vi "DDE2TCP_main.vi"() -> ()   [LabVIEW 2013]
uses:
  <vilib>/Utility/error.llb/DialogType.ctl
  _OpenG.lib/comparison.llb/Variant Changed__ogtk.vi
panel:
  in  "listen halted":bool caption="Listener gestoppt"
  in  "empty":refnum<k5>[](array[refnum]) caption="Leer"
  in  "empty 2":refnum<k5>[](array[refnum]) caption="Leer"
  out "Pfad":path
  out "String":string
  in  "Registerkarte":enum32{"MyDDE2TCP", "Data file", "Sim"}(tab)
  out "status":bool
  out "data":string="\r\n" caption="DDE Message"
  out "# of Connections":dbl caption="Client connections"
  in  "Port":u16=6341 caption="TCP Port"
  in  "stop":bool caption="Stopp"
  out "Azimuth":string caption="°"
  out "Elevation":string caption="°"
  out "Satellite Name":string
  out "Downlink Freq. Setpoint":string caption="Hz"
  out "Uplink Freq. Setpoint":string caption="Hz"
  out "Current JD [UTC]":dbl=2456800.0578935184 format="%#.15g"
  out "Unix time":dbl=1400757802.7173696 format="%#_13g"
  out "Time Stamp (UTC)":timestamp=timestamp(3483602602.7173696 s since 1904-01-01) format="%^<%.3X   %x>T"
  out "Current Modified JD [UTC]":dbl=2456800.0578935184 format="%#.15g"
  in  "Sampling interval":u32=250 caption="[ms]"
  in  "Save Controls":bool
  out "Tracking data":string
  out "Path of the saved data":path
  out "concatenated string":string
  in  "Radio Buttons":enum32{"Realtime", "Simulated time"}(radio)
  in  "Simulated time":timestamp
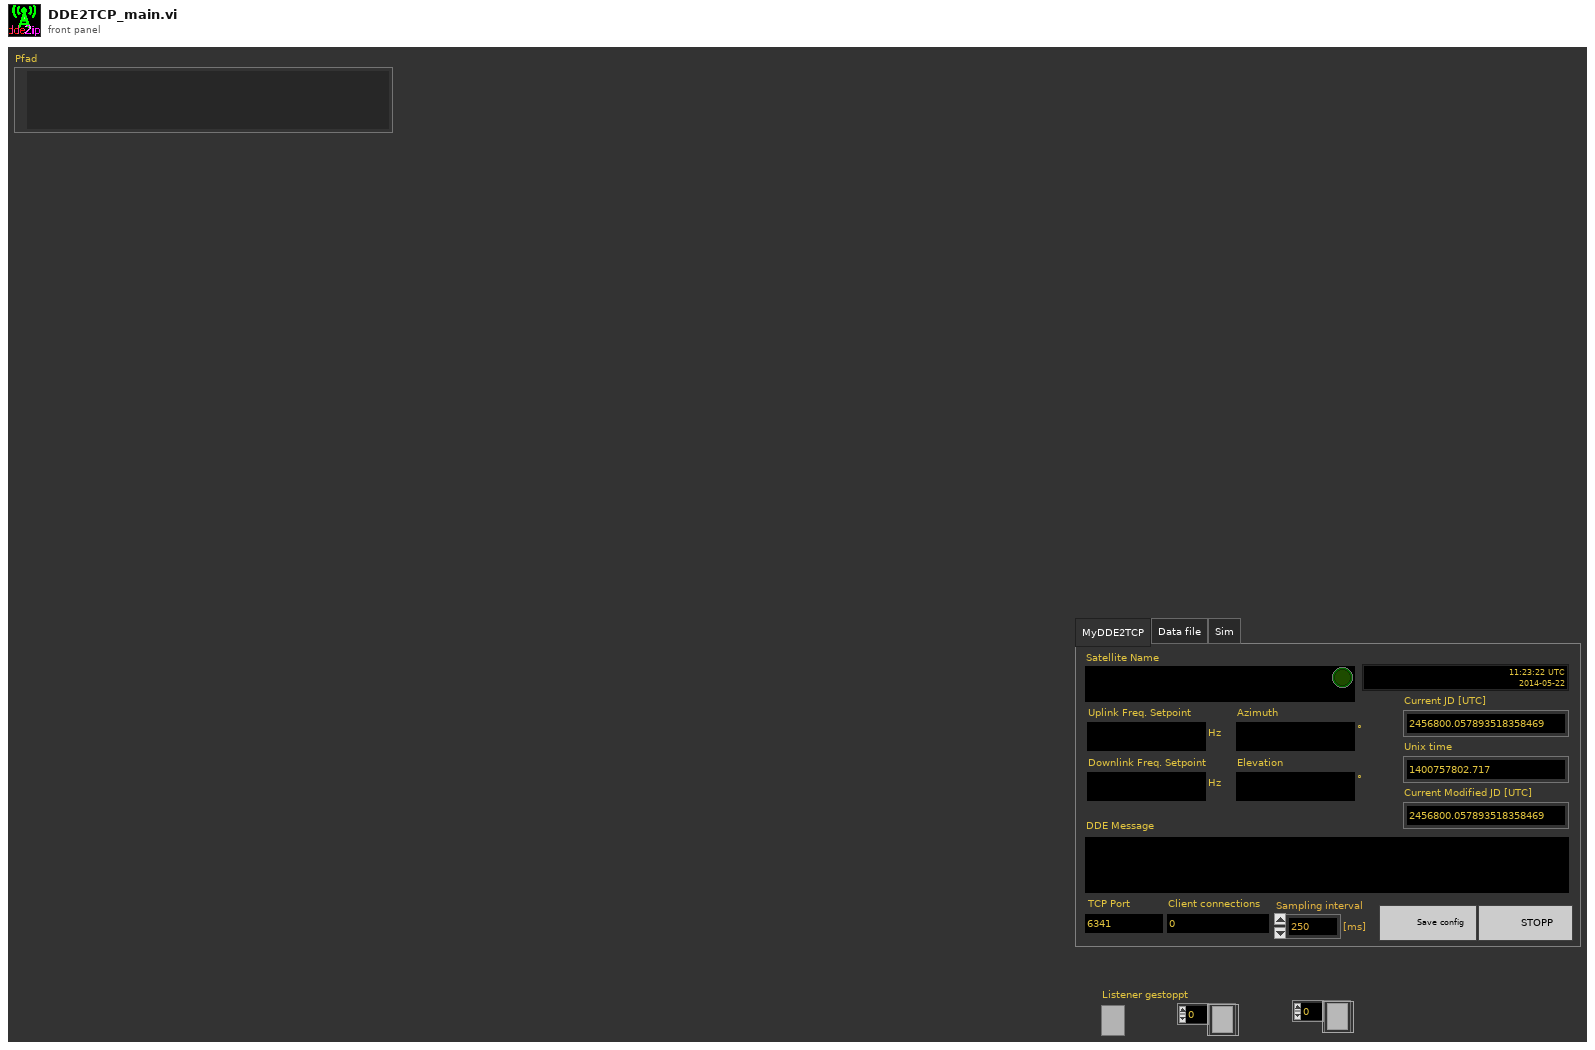
[diagram p1: front panel]
types:
  T1 = typedef "DialogType.ctl" = u16
  T2 = typedef "LVDateTimeRec.ctl" = cluster{"fractional second":dbl, "second":i32, "minute":i32, "hour":i32, "day of month":i32, "month":i32, "year":i32, "day of week":i32, "day of year":i32, "DST":i32}
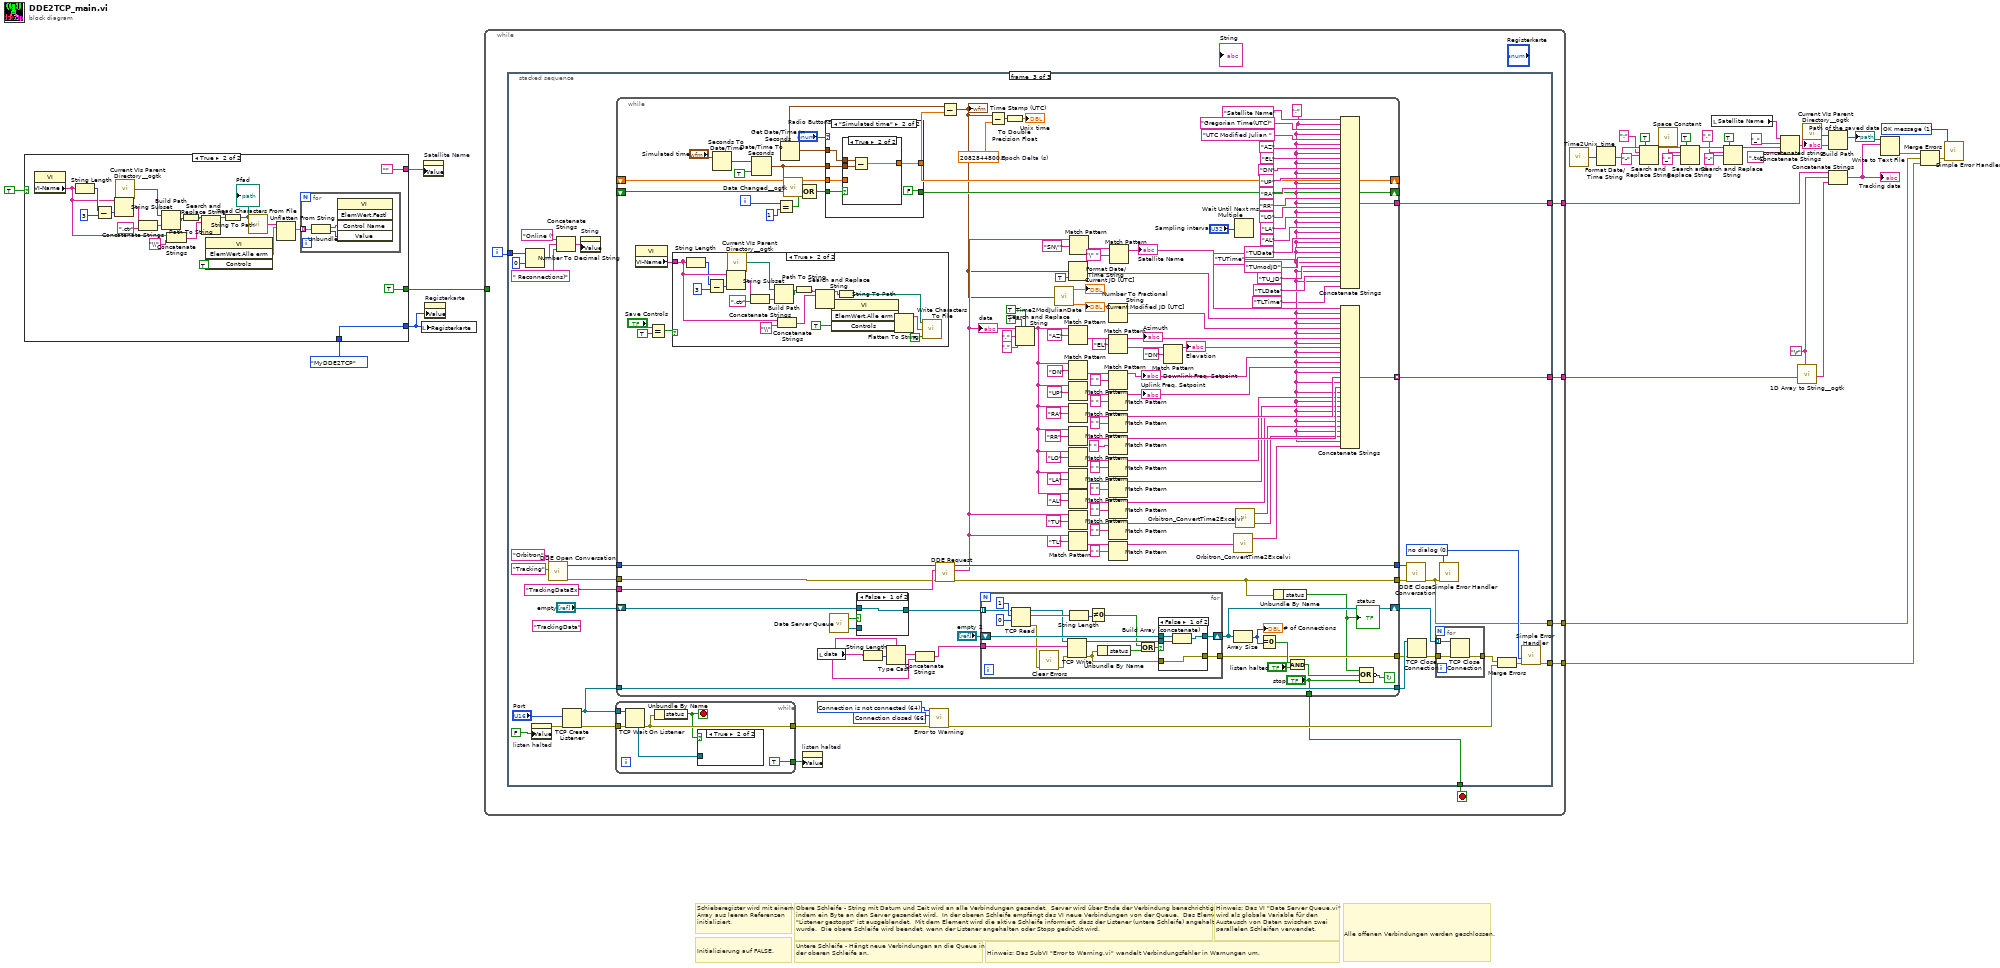
[diagram p0: block diagram]
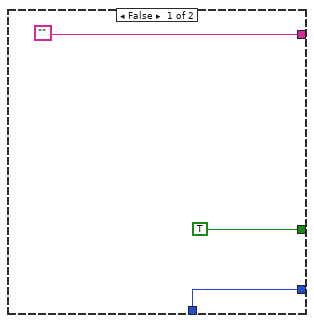
[diagram p2: hidden frame]
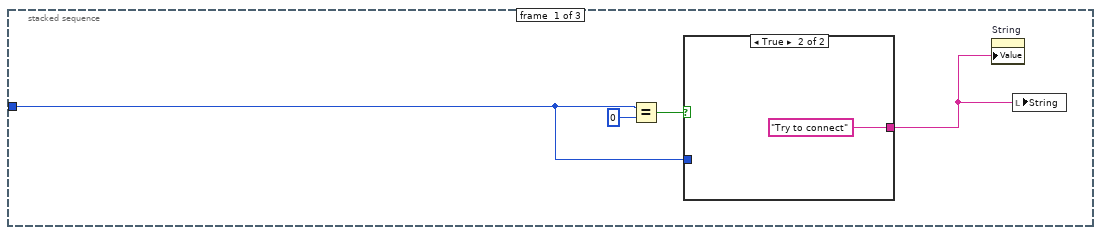
[diagram p3: hidden frame]
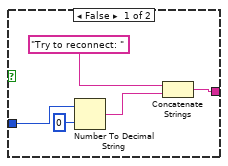
[diagram p4: hidden frame]
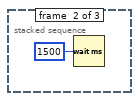
[diagram p5: hidden frame]
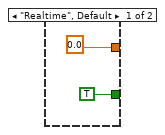
[diagram p7: hidden frame]
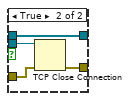
[diagram p9: hidden frame]
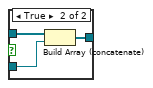
[diagram p10: hidden frame]
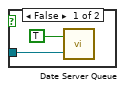
[diagram p11: hidden frame]
diagram:
  w8 = T1 1 items=["no dialog", "OK message", "continue or stop message", "OK message + warnings", "continue/stop + warnings"] ("type of dialog (OK msg:1)")
  w33 = "\r"
  # "Obere Schleife - String mit Datum und Zeit wird an alle Verbindungen gesendet.  Server wird über Ende der Verbindung benachrichtigt, indem ein Byte an den Server gesendet wird.  In der oberen Schleife empfängt das VI neue Verbindungen von der Queue.  Das Element \"Listener gestoppt\" ist ausgeblendet.  Mit dem Element wird die aktive Schleife informiert, dass der Listener (untere Schleife) angehalten wurde.  Die obere Schleife wird beendet, wenn der Listener angehalten oder Stopp gedrückt wird."
  # "Hinweis: Das VI \"Date Server Queue.vi\" wird als globale Variable für den Austausch von Daten zwischen zwei parallelen Schleifen verwendet."
  # "Hinweis: Das SubVI \"Error to Warning.vi\" wandelt Verbindungsfehler in Warnungen um."
  # "Schieberegister wird mit einem Array aus leeren Referenzen initialisiert."
  # "Untere Schleife - Hängt neue Verbindungen an die Queue in der oberen Schleife an."
  # "Initialisierung auf FALSE."
  # "Alle offenen Verbindungen werden geschlossen."
  n1 = case shown="True" TRUE {
    tunnel: [TRUE ("Radio Mode") TRUE ("Radio Mode")] -> w2
    tunnel: ["" ""] -> w3
    tunnel: [w36 w39] -> w4
    tunnel: enum32{"MyDDE2TCP", "Data file", "Sim"}."MyDDE2TCP" ("Registerkarte") -> [w36 w39]
    frame False {
    }
    frame True {
      n2 = property class="VI"() -> ("VI-Name"=w53:string)  [unwired: 2 in, 2 out]
      n3 = String Length(string=w53) -> (length=w54:i32)
      n4 = Subtract(x=w54, y=3) -> (x-y=w56:i32)
      n5 = String Subset(string=w53, length (rest)=w56) -> (substring=w57:string)  [unwired: 1 in]
      n6 = call "Current VIs Parent Directory__ogtk.vi"() -> ("Parent Directory (+ Relative)"=w42:path)  [unwired: 5 in]
      n7 = Concatenate Strings(w57, ".ctr" ("String")) -> (w59:string)
      n8 = Build Path(base path=w42, name or relative path=w59) -> (appended path=w48:path)
      n9 = Concatenate Strings(w53, "\\" ("string")) -> (w52:string)
      n10 = Path To String(path=w48) -> (string=w49:string)
      n11 = Search and Replace String(input string=w49, search string=w52) -> (result string=w50:string)  [unwired: 6 in, 3 out]
      n12 = invoke class="VI" method="ElemWert.Alle erm"("Controls"=TRUE ("controls")) -> ("Get All Control Values Variant"=w47:cluster{"Name":string, "Variant Data":variant}[])  [unwired: 3 in, 3 out]
      n13 = String To Path(string=w50) -> (path=w43:path)
      "Pfad" <- w43
      n14 = call <vilib>:"Read Characters From File.vi"("file path (dialog if empty)"=w43) -> ("character string"=w45:string)  [unwired: 5 in, 3 out]
      n15 = Unflatten From String(type=w47, binary string=w45) -> (value=w46:cluster{"Name":string, "Variant Data":variant}[])  [unwired: 3 in, 2 out]
      n16 = for {
        tunnel: w46 -> [w61] mode=indexing
        n17 = Unbundle(w61) -> ("Name"=w60:string, "Variant Data"=w62:variant)
        n18 = invoke class="VI" method="ElemWert.Festl"("Control Name"=w60, "Value"=w62) -> ()  [unwired: 3 in, 5 out]
      }
    }
  }
  n19 = local write "Registerkarte"(w4) -> ()
  n20 = property on="Satellite Name" class="Str"("Value"=w3) -> ()  [unwired: 2 in, 2 out]
  n21 = property on="Registerkarte" class="RKElem (strikt)"("Value"=w4) -> ()  [unwired: 2 in, 2 out]
  n22 = while {
    tunnel: [w68] -> w35
    tunnel: [w67] -> w34
    tunnel: [w64] -> w7
    tunnel: [w63] -> w6
    tunnel: w2 -> [_]
    i -> [w65]
    stop <- w66 stop-if-true
    n23 = stacked-sequence {
      tunnel: [_ _ w92] -> w68
      tunnel: [_ _ w91] -> w67
      tunnel: [_ _ w89] -> w66
      tunnel: w65 -> [w69 _ w84]
      tunnel: [_ _ w87] -> w64
      tunnel: [_ _ w86] -> w63
      frame #0 {
        n24 = Equal?(x=w69, y=0) -> (x = y?=w71:bool)
        n25 = case shown="True" w71 {
          tunnel: [w76 "Try to connect" ("String")] -> w70
          tunnel: w69 -> [w74 _]
          frame False {
            n26 = Number To Decimal String(number=w74, width (-)=i16 0) -> (decimal integer string=w75:string)
            n27 = Concatenate Strings("Try to reconnect: " ("String"), w75) -> (w76:string)
          }
          frame True {
          }
        }
        n28 = property on="String" class="Str"("Value"=w70) -> ()  [unwired: 2 in, 2 out]
        n29 = local write "String"(w70) -> ()
      }
      frame #1 {
        n30 = Wait (ms)(milliseconds to wait=u32 1500) -> ()  [unwired: 1 out]
      }
      frame #2 {
        w88 = T1 0 items=["no dialog", "OK message", "continue or stop message", "OK message + warnings", "continue/stop + warnings"] ("type of dialog (OK msg:1)")
        (unwired) "TrackingData" ("item")
        w104 = 66 items=["No Error", "Argument Error", "Memory Full", "Out of Zone", "End of File", "File Already Open", "Generic File IO Error", "File Not Found", "File Permission Error", "Disk Full", "Duplicate Path", "Too Many Files Open", "Not Enabled", "Resource File Not Found", "Cannot Add Resource", "Resource Not Found", "Image Not Found", "Image Memory Error", "Pen Does Not Exist", "Config Bad Type", "Config Token Not Found", "Config Parse Error", "Config Memory Error", "Bad External Code Format", "Bad External Code Offset", "External Code Not Present", "Null Window", "Destroy Window Mixup", "Null Menu", "Print Aborted", "Bad Print Record", "Print Driver Error", "Windows Error During Print", "Memory Error During Print", "Print Dialog Error", "Generic Print Error", "Invalid Device Refnum", "Device Not Found", "Device Parameter Error", "Device Unit Error", "Can't Open Device", "Device Call Aborted", "Generic Error", "Cancelled By User", "Object ID Too Low", "Object ID Too High", "Object Not In Heap", "Unknown Heap", "Bad DefProc ID", "DefProc Not In Table", "Message Out Of Range", "Null Method", "Unknown Message", "Manager Call Not Supported", "Bad address", "Connection In progress", "Connection timed out", "Connection is already in progress", "Network attribute not supported", "Network error", "Address in use", "System out of memory", "Connection aborted", "Connection refused", "Connection is not connected", "Connection is already connected", "Connection closed", "Initialize error (interapplication manager)", "Bad occurrence", "Wait on unbound occurrence handler", "Occurrence queue overflow", "Bad path", "Semaphore not signaled", "Unrecognized type (interapplication manager)"] ("2nd Error to Convert")
        w105 = 64 items=["No Error", "Argument Error", "Memory Full", "Out of Zone", "End of File", "File Already Open", "Generic File IO Error", "File Not Found", "File Permission Error", "Disk Full", "Duplicate Path", "Too Many Files Open", "Not Enabled", "Resource File Not Found", "Cannot Add Resource", "Resource Not Found", "Image Not Found", "Image Memory Error", "Pen Does Not Exist", "Config Bad Type", "Config Token Not Found", "Config Parse Error", "Config Memory Error", "Bad External Code Format", "Bad External Code Offset", "External Code Not Present", "Null Window", "Destroy Window Mixup", "Null Menu", "Print Aborted", "Bad Print Record", "Print Driver Error", "Windows Error During Print", "Memory Error During Print", "Print Dialog Error", "Generic Print Error", "Invalid Device Refnum", "Device Not Found", "Device Parameter Error", "Device Unit Error", "Can't Open Device", "Device Call Aborted", "Generic Error", "Cancelled By User", "Object ID Too Low", "Object ID Too High", "Object Not In Heap", "Unknown Heap", "Bad DefProc ID", "DefProc Not In Table", "Message Out Of Range", "Null Method", "Unknown Message", "Manager Call Not Supported", "Bad address", "Connection In progress", "Connection timed out", "Connection is already in progress", "Network attribute not supported", "Network error", "Address in use", "System out of memory", "Connection aborted", "Connection refused", "Connection is not connected", "Connection is already connected", "Connection closed", "Initialize error (interapplication manager)", "Bad occurrence", "Wait on unbound occurrence handler", "Occurrence queue overflow", "Bad path", "Semaphore not signaled", "Unrecognized type (interapplication manager)"] ("1st Error to Convert")
        n31 = Number To Decimal String(number=w84, width (-)=i16 0) -> (decimal integer string=w85:string)
        n32 = property on="listen halted" class="Bool. (strikt)"("Value"=FALSE) -> (error out=w101:errorcluster)  [unwired: 2 in, 1 out]
        n33 = call <vilib>:"DDE Open Conversation.vi"("topic"="Tracking" ("Topic"), "service"="Orbitron" ("Service")) -> ("error out"=w95:errorcluster, "conversation refnum"=w96:u32)  [unwired: 6 in]
        n34 = Concatenate Strings("Online (" ("String"), w85, " Reconnections)") -> (w81:string)
        n35 = TCP Create Listener(8:w101, 10:"Port") -> (0:w110:errorcluster, 3:w108:refnum<k5>)  [unwired: 4 out]
        n36 = property on="String" class="Str"("Value"=w81) -> ()  [unwired: 2 in, 2 out]
        n37 = while "Listen loop.  Append new connections to a synchronized queue." {
          tunnel: w108 -> [w308]
          tunnel: w110 -> [w309]
          tunnel: [w306] -> w106
          tunnel: [TRUE] -> w107
          stop <- w305 stop-if-true
          n38 = TCP Wait On Listener(8:w309, 11:w308) -> (0:w306:errorcluster, 4:w307:refnum<k5>)  [unwired: 5 out]
          n39 = Unbundle By Name(w306) -> ("status"=w305:bool)
          n40 = case shown="True" w305 {
            tunnel: w307 -> [w310 _]
            frame False {
              n41 = call "Date Server Queue.vi"("new value"=w310, "set queue? (F: de-queue)"=TRUE) -> ()  [unwired: 2 out]
            }
            frame True {
            }
          }
        }
        n42 = while {
          shift-left: "empty" -> [w242]
          shift-right: [w239] -> w112
          tunnel: w108 -> [w234]
          tunnel: [w234] -> w109
          tunnel: [w233] -> w100
          tunnel: w96 -> [w227]
          tunnel: w95 -> [w226]
          tunnel: "TrackingDataEx" ("item") -> [w228]
          tunnel: [w225] -> w94
          tunnel: [w121] -> w93
          tunnel: [w212] -> w92 mode=indexing
          tunnel: [w200] -> w91
          shift-right: [w147] -> _
          shift-left: _ -> [w148]
          shift-right: [w146] -> _
          shift-left: _ -> [w145]
          tunnel: ["stop"] -> w89
          i -> [w144]
          stop <- w120 continue-if-true
          w142 = 2082844800.0  # Epoch Delta (s)
          w124 = ";"
          n43 = property class="VI"() -> ("VI-Name"=w118:string)  [unwired: 2 in, 2 out]
          n44 = Equal?(x="Save Controls", y=TRUE) -> (x = y?=w117:bool)
          n45 = case shown="True" w117 {
            tunnel: w118 -> [_ w262]
            frame False {
            }
            frame True {
              n46 = String Length(string=w262) -> (length=w256:i32)
              n47 = Subtract(x=w256, y=3) -> (x-y=w258:i32)
              n48 = String Subset(string=w262, length (rest)=w258) -> (substring=w259:string)  [unwired: 1 in]
              n49 = call "Current VIs Parent Directory__ogtk.vi"() -> ("Parent Directory (+ Relative)"=w246:path)  [unwired: 5 in]
              n50 = Concatenate Strings(w259, ".ctr" ("String")) -> (w261:string)
              n51 = Build Path(base path=w246, name or relative path=w261) -> (appended path=w251:path)
              n52 = Concatenate Strings(w262, "\\" ("string")) -> (w255:string)
              n53 = Path To String(path=w251) -> (string=w252:string)
              n54 = Search and Replace String(input string=w252, search string=w255) -> (result string=w253:string)  [unwired: 6 in, 3 out]
              n55 = invoke class="VI" method="ElemWert.Alle erm"("Controls"=TRUE ("controls")) -> ("Get All Control Values Variant"=w249:cluster{"Name":string, "Variant Data":variant}[])  [unwired: 3 in, 3 out]
              n56 = String To Path(string=w253) -> (path=w245:path)
              n57 = Flatten To String(anything=w249) -> (data string=w248:string)  [unwired: 3 in, 2 out]
              n58 = call <vilib>:"Write Characters To File.vi"("append to file? (new file:F)"=FALSE, "character string"=w248, "file path (dialog if empty)"=w245) -> ()  [unwired: 2 in, 1 out]
            }
          }
          n59 = Seconds To Date/Time(time stamp (now)="Simulated time") -> (date time rec=w139:T2)  [unwired: 1 in]
          n60 = Date/Time To Seconds(1:TRUE ("is UTC (F)"), 2:w139) -> (0:w136:timestamp)
          n61 = Equal?(x=w144, y=1) -> (x = y?=w153:bool)
          n62 = Get Date/Time In Seconds() -> (seconds since 1Jan1904=w151:timestamp)
          n63 = call-poly "Data Changed__ogtk.vi"("Variant"=w136) -> ("Changed"=w150:bool)
          n64 = Compound Arithmetic op=OR(w150, w145, w153) -> (w149:bool)
          n65 = local read "data"() -> (w232:string)
          n66 = case shown="\"Simulated time\"" "Radio Buttons" {
            tunnel: [0.0 w270] -> w147
            tunnel: w148 -> [_ w269]
            tunnel: w149 -> [_ w268]
            tunnel: w151 -> [_ w267]
            tunnel: w136 -> [_ w266]
            tunnel: [TRUE FALSE] -> w146
            frame "Realtime", Default {
            }
            frame "Simulated time" {
              n67 = case shown="True" w268 {
                tunnel: [w271 w272] -> w270
                tunnel: w269 -> [w271 _]
                tunnel: w267 -> [_ w274]
                tunnel: w266 -> [_ w273]
                frame False {
                }
                frame True {
                  n68 = Subtract(x=w274, y=w273) -> (x-y=w272:dbl)
                }
              }
            }
          }
          n69 = call "Date Server Queue.vi"() -> ("value"=w244:refnum<k5>, "valid?"=w243:bool)  [unwired: 2 in]
          n70 = case shown="False" w243 {
            tunnel: w244 -> [_ w303]
            tunnel: w242 -> [w300 w302]
            tunnel: [w300 w301] -> w241
            frame False {
            }
            frame True {
              n71 = Build Array (concatenate)(w302, w303) -> (w301:refnum<k5>[])
            }
          }
          n72 = String Length(string=w232) -> (length=w230:i32)
          n73 = Type Cast(type=w232, x=w230) -> (*(type *) &x=w231:string)
          n74 = Concatenate Strings(w231, w232) -> (w229:string)
          n75 = call <vilib>:"DDE Request.vi"("error in (no error)"=w226, "item"=w228, "conversation refnum in"=w227) -> ("error out"=w121:errorcluster, "data"=w159:string, "conversation refnum out"=w225:u32)  [unwired: 4 in]
          "data" <- w159
          n76 = Subtract(x=w151, y=w147) -> (x-y=w140:timestamp)
          "Time Stamp (UTC)" <- w140
          n77 = for {
            tunnel: w241 -> [w281] mode=indexing
            shift-right: [w288] -> w239
            shift-left: "empty 2" -> [w290]
            tunnel: w229 -> [w291]
            tunnel: [w275] -> w233
            n78 = TCP Read(connection ID=w281, bytes to read=1, 9:0) -> (connection ID out=w280:refnum<k5>, data out=w285:string, error out=w277:errorcluster)  [unwired: 1 in, 1 out]
            n79 = call <vilib>:"Clear Errors.vi"("error in (no error)"=w277) -> ("error out"=w276:errorcluster)  [unwired: 6 out]
            n80 = TCP Write(connection ID=w280, data in=w291, error in (no error)=w276) -> (connection ID out=w289:refnum<k5>, error out=w278:errorcluster)  [unwired: 2 out]
            n81 = String Length(string=w285) -> (length=w284:i32)
            n82 = Not Equal To 0?(x=w284) -> (x != 0?=w282:bool)
            n83 = Unbundle By Name(w278) -> ("status"=w279:bool)
            n84 = Or(x=w282, y=w279) -> (x .or. y?=w283:bool)
            n85 = case shown="False" w283 {
              tunnel: w290 -> [w295 w299]
              tunnel: w289 -> [w294 w298]
              tunnel: [w293 w299] -> w288
              tunnel: w278 -> [w292 w297]
              tunnel: [w292 w296] -> w275
              frame False {
                n86 = Build Array (concatenate)(w295, w294) -> (w293:refnum<k5>[])
              }
              frame True {
                n87 = TCP Close Connection(connection ID=w298, error in (no error)=w297) -> (error out=w296:errorcluster)  [unwired: 2 out]
              }
            }
          }
          n88 = Subtract(x=w140, y=w142) -> (x-y=w143:timestamp)
          n89 = To Double Precision Float(number=w143) -> (double precision float=→"Unix time":dbl)
          n90 = Search and Replace String(replace all?=TRUE ("replace all? (F)"), case sensitive?=TRUE ("ignore case? (F)"), input string=w159, search string=".", replace string="," ("replace string (\"\")")) -> (result string=w131:string)  [unwired: 3 in, 3 out]
          n91 = call "Time2ModJulianDate.vi"("Time of Propagation (UTC)  2"=w140) -> ("ModifiedJulian"=w210:dbl, "JD"=→"Current JD [UTC]":dbl)  [unwired: 4 in, 2 out]
          "Current Modified JD [UTC]" <- w210
          n92 = Match Pattern(string=w131, regular expression="AZ" ("Regulärer Ausdruck")) -> (after substring=w224:string)  [unwired: 1 in, 3 out]
          n93 = Match Pattern(string=w131, regular expression="DN" ("Regulärer Ausdruck")) -> (after substring=w219:string)  [unwired: 1 in, 3 out]
          n94 = Match Pattern(string=w131, regular expression="UP" ("Regulärer Ausdruck")) -> (after substring=w220:string)  [unwired: 1 in, 3 out]
          n95 = Match Pattern(string=w131, regular expression="RA" ("Regulärer Ausdruck")) -> (after substring=w180:string)  [unwired: 1 in, 3 out]
          n96 = Match Pattern(string=w131, regular expression="RR" ("Regulärer Ausdruck")) -> (after substring=w172:string)  [unwired: 1 in, 3 out]
          n97 = Match Pattern(string=w131, regular expression="LO" ("Regulärer Ausdruck")) -> (after substring=w175:string)  [unwired: 1 in, 3 out]
          n98 = Match Pattern(string=w131, regular expression="LA" ("Regulärer Ausdruck")) -> (after substring=w169:string)  [unwired: 1 in, 3 out]
          n99 = Match Pattern(string=w131, regular expression="AL" ("Regulärer Ausdruck")) -> (after substring=w168:string)  [unwired: 1 in, 3 out]
          n100 = Match Pattern(string=w159, regular expression="TU" ("Regulärer Ausdruck")) -> (after substring=w165:string)  [unwired: 1 in, 3 out]
          n101 = Match Pattern(string=w159, regular expression="TL" ("Regulärer Ausdruck")) -> (after substring=w162:string)  [unwired: 1 in, 3 out]
          n102 = Format Date/Time String(seconds (now)=w140, UTC format=TRUE) -> (date/time string=w214:string)  [unwired: 1 in]
          n103 = Match Pattern(string=w159, regular expression="SN\"" ("Regulärer Ausdruck")) -> (after substring=w216:string)  [unwired: 1 in, 3 out]
          n104 = Match Pattern(string=w224, regular expression="EL" ("Regulärer Ausdruck")) -> (before substring=w203:string, after substring=w223:string)  [unwired: 1 in, 2 out]
          "Azimuth" <- w203
          n105 = Match Pattern(string=w219, regular expression=" " ("Regulärer Ausdruck")) -> (before substring=w202:string)  [unwired: 1 in, 3 out]
          "Downlink Freq. Setpoint" <- w202
          n106 = Match Pattern(string=w220, regular expression=" " ("Regulärer Ausdruck")) -> (before substring=w201:string)  [unwired: 1 in, 3 out]
          "Uplink Freq. Setpoint" <- w201
          n107 = Match Pattern(string=w180, regular expression=" " ("Regulärer Ausdruck")) -> (before substring=w158:string)  [unwired: 1 in, 3 out]
          n108 = Match Pattern(string=w172, regular expression=" " ("Regulärer Ausdruck")) -> (before substring=w157:string)  [unwired: 1 in, 3 out]
          n109 = Match Pattern(string=w175, regular expression=" " ("Regulärer Ausdruck")) -> (before substring=w156:string)  [unwired: 1 in, 3 out]
          n110 = Match Pattern(string=w169, regular expression=" " ("Regulärer Ausdruck")) -> (before substring=w155:string)  [unwired: 1 in, 3 out]
          n111 = Match Pattern(string=w168, regular expression=" " ("Regulärer Ausdruck")) -> (before substring=w129:string)  [unwired: 1 in, 3 out]
          n112 = Match Pattern(string=w165, regular expression=" " ("Regulärer Ausdruck")) -> (before substring=w135:string)  [unwired: 1 in, 3 out]
          n113 = Match Pattern(string=w162, regular expression=" " ("Regulärer Ausdruck")) -> (before substring=w133:string)  [unwired: 1 in, 3 out]
          n114 = Number To Fractional String(number=w210) -> (F-format string=w204:string)  [unwired: 3 in]
          n115 = Match Pattern(string=w216, regular expression="\" " ("Regulärer Ausdruck")) -> (before substring=w198:string)  [unwired: 1 in, 3 out]
          "Satellite Name" <- w198
          n116 = Match Pattern(string=w223, regular expression="DN" ("Regulärer Ausdruck")) -> (before substring=w195:string)  [unwired: 1 in, 3 out]
          "Elevation" <- w195
          n117 = Array Size(array=w239) -> (size(s)=w237:i32)
          "# of Connections" <- w237
          n118 = call "Orbitron_ConvertTime2Excelvi.vi"("OrbitronTimeDateString"=w133) -> ("DateTime"=w127:string)  [unwired: 1 in, 1 out]
          n119 = Wait Until Next ms Multiple(millisecond multiple="Sampling interval") -> ()  [unwired: 1 out]
          n120 = call "Orbitron_ConvertTime2Excelvi.vi"("OrbitronTimeDateString"=w135) -> ("JD&ModJD"=w128:string, "DateTime"=w134:string)  [unwired: 1 in]
          n121 = Equal To 0?(x=w237) -> (x = 0?=w238:bool)
          n122 = Unbundle By Name(w121) -> ("status"=w119:bool)
          "status" <- w119
          n123 = And(x=w238, y="listen halted") -> (x .and. y?=w236:bool)
          n124 = Concatenate Strings(w198, w124, w214, w124, w204, w124, w203, w124, w195, w124, w202, w124, w201, w124, w158, w124, w157, w124, w156, w124, w155, w124, w129, w124, w134, w124, w128, w124, w127) -> (w212:string)
          n125 = Concatenate Strings("Satellite Name" ("String"), w124, "Gregorian Time(UTC)" ("String"), w124, "UTC Modified Julian " ("String"), w124, "AZ" ("Regulärer Ausdruck"), w124, "EL" ("Regulärer Ausdruck"), w124, "DN" ("Regulärer Ausdruck"), w124, "UP" ("Regulärer Ausdruck"), w124, "RA" ("Regulärer Ausdruck"), w124, "RR" ("Regulärer Ausdruck"), w124, "LO" ("Regulärer Ausdruck"), w124, "LA" ("Regulärer Ausdruck"), w124, "AL" ("Regulärer Ausdruck"), w124, "TUDate" ("Regulärer Ausdruck"), w124, "TUTime" ("Regulärer Ausdruck"), w124, "TUmodJD" ("Regulärer Ausdruck"), w124, "TU_JD" ("Regulärer Ausdruck"), w124, "TLDate" ("Regulärer Ausdruck"), w124, "TLTime" ("Regulärer Ausdruck")) -> (w200:string)
          n126 = Compound Arithmetic op=OR(w119, w236, "stop") -> (invert w120:bool)
        }
        n127 = property on="listen halted" class="Bool. (strikt)"("Value"=w107) -> ()  [unwired: 2 in, 2 out]
        n128 = call <vilib>:"Error to Warning.vi"("1st Error to Convert"=w105, "2nd Error to Convert"=w104, "error in"=w106) -> ("warning out"=w98:errorcluster)  [unwired: 2 in, 10 out]
        n129 = call <vilib>:"DDE Close Conversation.vi"("error in (no error)"=w93, "conversation refnum"=w94) -> ("error out"=w86:errorcluster)  [unwired: 7 in]
        n130 = TCP Close Connection(connection ID=w109, error in (no error)=w100) -> (error out=w99:errorcluster)  [unwired: 2 out]
        n131 = for {
          tunnel: w112 -> [w314] mode=indexing
          tunnel: [w313] -> w103
          tunnel: w99 -> [w312]
          n132 = TCP Close Connection(connection ID=w314, error in (no error)=w312) -> (error out=w313:errorcluster)  [unwired: 2 out]
        }
        n133 = call <vilib>:"Simple Error Handler.vi"("type of dialog (OK msg:1)"=w88, "error in (no error)"=w86) -> ()  [unwired: 8 out]
        n134 = Merge Errors(w103, w98) -> (w87:errorcluster)
        n135 = call <vilib>:"Simple Error Handler.vi"("type of dialog (OK msg:1)"=w88, "error in (no error)"=w87) -> ()  [unwired: 8 out]
      }
    }
  }
  n136 = call "Time2Unix_time.vi"() -> ("seconds since 1Jan1904"=w26:timestamp)  [unwired: 10 in, 1 out]
  n137 = Format Date/Time String(seconds (now)=w26) -> (date/time string=w25:string)  [unwired: 2 in]
  n138 = Search and Replace String(replace all?=TRUE ("replace all? (F)"), input string=w25, search string=":", replace string="-" ("replace string (\"\")")) -> (result string=w19:string)  [unwired: 4 in, 3 out]
  n139 = call <vilib>:"Space Constant.vi"() -> ("String"=w18:string)
  n140 = Search and Replace String(replace all?=TRUE ("replace all? (F)"), input string=w19, search string=w18, replace string="_" ("replace string (\"\")")) -> (result string=w15:string)  [unwired: 4 in, 3 out]
  n141 = local read "Satellite Name"() -> (w12:string)
  n142 = Search and Replace String(replace all?=TRUE ("replace all? (F)"), input string=w15, search string=",", replace string="-" ("replace string (\"\")")) -> (result string=w14:string)  [unwired: 4 in, 3 out]
  n143 = Concatenate Strings(w12, "_", w14, ".txt") -> (w29:string)
  "concatenated string" <- w29
  n144 = call "1D Array to String__ogtk.vi"("delimiter (Tab)"=w33, "Array of Strings"=w35) -> ("delimited string"=w32:string)  [unwired: 9 in]
  n145 = call "Current VIs Parent Directory__ogtk.vi"() -> ("Parent Directory (+ Relative)"=w30:path)  [unwired: 5 in]
  n146 = Concatenate Strings(w34, w33, w32) -> (w31:string)
  "Tracking data" <- w31
  n147 = Build Path(base path=w30, name or relative path=w29) -> (appended path=w28:path)
  "Path of the saved data" <- w28
  n148 = Write to Text File(file (use dialog)=w28, text=w31) -> (error out=w10:errorcluster)  [unwired: 2 in, 2 out]
  n149 = Merge Errors(w10, w6, w7) -> (w9:errorcluster)
  n150 = call <vilib>:"Simple Error Handler.vi"("type of dialog (OK msg:1)"=w8, "error in (no error)"=w9) -> ()  [unwired: 8 out]
